vi "bmp085_init.vi"(4 "Allow multiple opens?":bool=TRUE, 6 "I2C User Configuration":T1, 7 "Oversampling Setting (oss)":T3(ring), 8 "error in (no error)":errorcluster, 10 "Slave Address (7-bit)":u8=119 format="%.0x", 11 "Channel Name":tag="A/I2C") -> (0 "error out":errorcluster, 3 "BMP085 (GY-65) out":refnum<class "BMP085 (GY-65).lvclass">)   [LabVIEW 2015, in "BMP085 (RT).lvlib" / "BMP085 (GY-65).lvclass"]
uses:
  BMP085 (GY-65).lvclass
  <vilib>/myRIO/Instrument Drivers/Onboard IO/I2C/typedefs/I2C User Configuration.ctl
  <vilib>/myRIO/Instrument Drivers/Onboard IO/I2C/typedefs/I2C Transfer Rate.ctl
  BMP085 (GY-65).lvclass/BMP085 (GY-65).ctl
  <vilib>/Utility/error.llb/Error Cluster From Error Code.vi
  <vilib>/myRIO/Common/Instrument Driver Framework/myRIO v1.0/I2C/vis/myRIO v1.0 Configure I2C.vi
  <vilib>/myRIO/Instrument Drivers/Onboard IO/I2C/I2C.lvlib
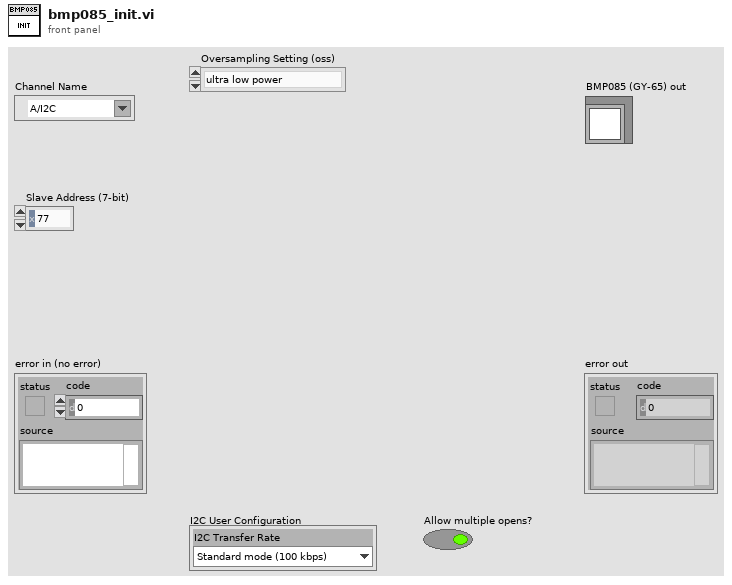
[diagram p1: front panel]
types:
  T1 = typedef "I2C.lvlib/I2C User Configuration.ctl" = cluster{"I2C Transfer Rate":T2}
  T2 = typedef "I2C.lvlib/I2C Transfer Rate.ctl" = enum16{"Standard mode (100 kbps)", "Fast mode (400 kbps)"}
  T3 = enum8{"ultra low power", "standard", "high resolution", "ultra high resolution"}
  T4 = typedef "I2C.lvlib/I2C Reference.ctl" = cluster{"myRIO Reference":T5, "I2C Channels Enum":T9, "I2C Configuration":T10}
  T5 = typedef "myRIO Generic Hardware Reference.ctl" = cluster{"myRIO Model":T6, "myRIO Hardware Reference":T7}
  T6 = typedef "Hardware Version Enum.ctl" = enum16{"Unknown", "myRIO-1900", "myRIO-1950", "roboRIO"}
  T7 = typedef "myRIO v1.0 Reference.ctl" = cluster{"Generic FPGA Reference":T8, "Allow multiple opens":bool}
  T8 = typedef "Generic FPGA Reference.ctl" = refnum<k20>
  T9 = typedef "I2C Channels Enum.ctl" = enum16{"Not Connected", "A/I2C", "B/I2C", "I2C/I2C"}
  T10 = typedef "I2C.lvlib/I2C Configuration.ctl" = cluster{"I2C Transfer Rate":T2}
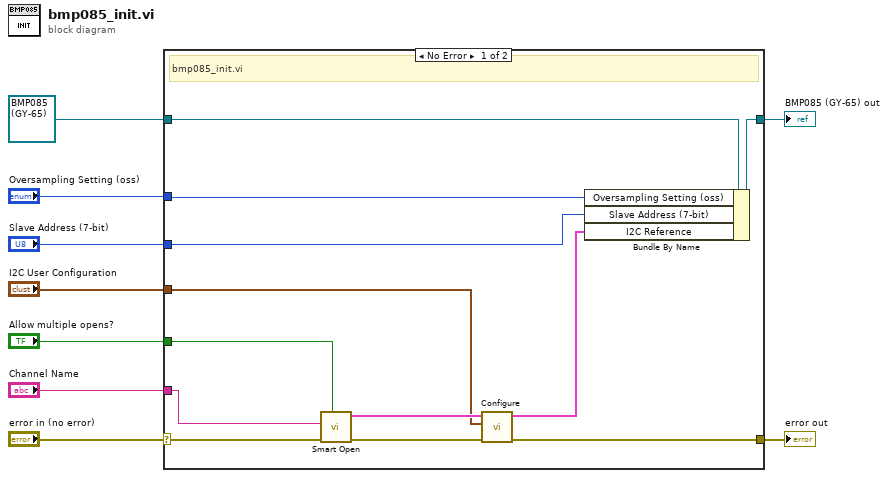
[diagram p0: block diagram]
diagram:
  n1 = case shown="No Error" "error in (no error)" {
    selector: "error in (no error)" -> [w19 w23]
    tunnel: [w18 w23] -> w8
    tunnel: [w15 w22] -> w6
    tunnel: refnum<class "BMP085 (GY-65).lvclass"> refnum ("BMP085 (GY-65) in") -> [w16 w22]
    tunnel: "Channel Name" -> [w17 _]
    tunnel: "Slave Address (7-bit)" -> [w13 _]
    tunnel: "Oversampling Setting (oss)" -> [w12 _]
    tunnel: "I2C User Configuration" -> [w11 _]
    tunnel: "Allow multiple opens?" -> [w10 _]
    frame No Error {
      # "bmp085_init.vi"
      n2 = call <vilib>:"Smart Open.vi"("Allow multiple opens?"=w10, "error in (no error)"=w19, "Channel Name"=w17) -> ("error out"=w20:errorcluster, "I2C Ref Out"=w21:T4)  [unwired: 7 in]
      n3 = call <vilib>:"Configure.vi"("error in (no error)"=w20, "I2C User Configuration"=w11, "I2C Ref In"=w21) -> ("error out"=w18:errorcluster, "I2C Ref Out"=w14:T4)  [unwired: 7 in]
      n4 = Bundle By Name(cluster=w16, "Oversampling Setting (oss)"=w12, "Slave Address (7-bit)"=w13, "I2C Reference"=w14) -> (w15:refnum<class "BMP085 (GY-65).lvclass">)
    }
    frame Error {
    }
  }
  "error out" <- w8
  "BMP085 (GY-65) out" <- w6
